vi "LAC Cmd121_ZOOM.vi"(6 "R/W (F:Read)":bool, 7 "timeout(ms)":u32=500, 8 "error in":errorcluster, 9 "zoom_val":T1={"mode"=enum."Fixed value", "Fixed_val"=enum."x4", "Input_val"=1.1}, 11 "VISA name in":refnum<visa-resource-name>) -> (0 "error out":errorcluster, 1 "readout":string, 3 "VISA name out":refnum<visa-resource-name>)   [LabVIEW 2018]
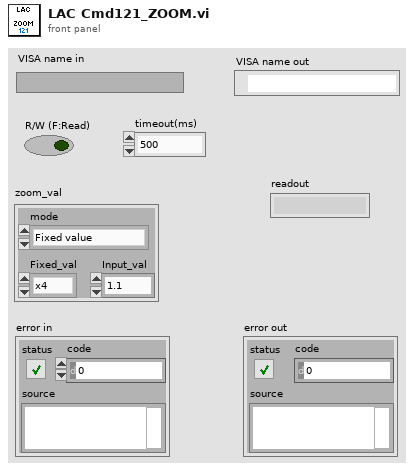
[diagram p1: front panel]
types:
  T1 = cluster{"mode":enum16{"OFF", "Fixed value", "Input value"}, "Fixed_val":enum16{"x2", "x4", "x8"}, "Input_val":dbl}
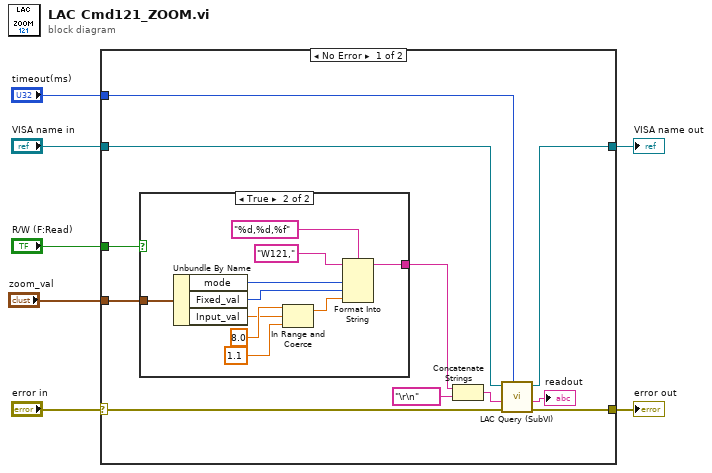
[diagram p0: block diagram]
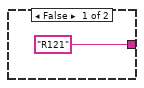
[diagram p2: hidden frame]
diagram:
  n1 = case shown="No Error" "error in" {
    selector: "error in" -> [w14 w31]
    tunnel: "VISA name in" -> [w16 w30]
    tunnel: [w18 w30] -> w6
    tunnel: [w17 w31] -> w5
    tunnel: "timeout(ms)" -> [w15 _]
    tunnel: "R/W (F:Read)" -> [w9 _]
    tunnel: "zoom_val" -> [w8 _]
    frame No Error {
      n2 = case shown="True" w9 {
        tunnel: ["R121" ("string") w27] -> w10
        tunnel: w8 -> [_ w23]
        frame False {
        }
        frame True {
          n3 = Unbundle By Name(w23) -> ("mode"=w20:enum16{"OFF", "Fixed value", "Input value"}, "Fixed_val"=w21:enum16{"x2", "x4", "x8"}, "Input_val"=w22:dbl)
          n4 = In Range and Coerce(upper limit=8.0, x=w22, lower limit=1.1) -> (coerced(x)=w26:dbl)  [unwired: 1 out]
          n5 = Format Into String(format string="%d,%d,%f", initial string="W121," ("string"), w20, w21, w26) -> (resulting string=w27:string)  [unwired: 1 in, 1 out]
        }
      }
      n6 = Concatenate Strings(w10, "\r\n" ("write buffer")) -> (w12:string)
      n7 = call "LAC Query (SubVI).vi"("timeout(ms)"=w15, "error in"=w14, "Command"=w12, "VISA name in"=w16) -> ("error out"=w17:errorcluster, "read buffer"=→"readout":string, "VISA name out"=w18:refnum<visa-resource-name>)  [unwired: 5 in]
    }
    frame Error {
    }
  }
  "VISA name out" <- w6
  "error out" <- w5
